vi "Add mppt data to log file.vi"(0 "Experiment Indicator":string, 1 "Cell details cluster":T3={"Cell Position"=16, "Cell Label"="", "Pixel to measure"=0, "Area (cm^2)"=0.126, "Variable"="", "Variable value"="", "Scan settings in queue"=0, "Light or dark"="", "Measurement Type"=""} {"Pixel to measure" items=["All", "1", "2", "3", "4", "5", "6", "7", "8"]}, 3 "Intensity (no. of suns)":string, 4 "mppt folder path":path, 5 "mppt file path":path, 7 "Scan settings":T1={"J-V scan"=TRUE, "J-t scan"=FALSE, "Min voltage (V)"=0.0, "Max voltage (V)"=1.4, "Step (V)"=0.01, "Measurement delay (ms)"=10.0, "1st scan FB-SC"=TRUE, "Inverted structure"=FALSE, "Stabilisation time (s)"=0.0, "Stabilisation mode"=0, "Stabilisation value (V or A) "=0.0, "Step time (s)"=1.0, "Integration time"=0, "Repeat light scans"=FALSE, "Stabilisation in the dark?"=FALSE, "J-t Min (V)"=0.0, "J-t Max (V)"=1.4, "J-t Step (V)"=0.01, "Max. power stabilisation"=FALSE, "J-t 1st scan FB-SC"=TRUE, "J-t Inverted structure"=FALSE, "Max power tracking"=FALSE, "Vmp (V)"=0.7, "Total stabilisation time (s)"=100.0, "J-t best pixel only"=0, "Max power best pixel only"=0, "Vmp from J-V scan"=FALSE, "Intensity dependence"=FALSE, "P dep best pixel only"=0, "External quantum efficiency"=FALSE, "EQE best pixel only"=0, "WL min (nm)"=300.0, "WL max (nm)"=900.0, "WL step (nm)"=5.0, "Wait (ms)"=100.0, "No. of repeat scans"=2.0, "Only repeat for best pixel"=0, "Chopper Freq.  (Hz)"=90.0, "Time Constant (s)"=2.0, "Stabilisation time step (s)"=1.0, "Illumination conditions"=2, "Scan rate min (V/s)"=0.1, "Scan rate max (V/s)"=1.0, "No. of scan rate steps"=1.0, "Scan rate voltage step priority"=FALSE, "Scan rate measurement delay priority"=FALSE, "J-t Illumination conditions"=0, "White bias  (no. of suns)"=200.0, "Max P stab. Specific voltage"=FALSE} {"J-t Illumination conditions" items=["Light only", "Dark only", "Light then dark", "Dark then light"]; "No. of scan rate steps" min=1.0 step=1.0; "Illumination conditions" items=["Light only", "Dark only", "Light then dark", "Dark then light", "Light then dark then light", "Dark then light then dark"]; "Time Constant (s)" items=["0.003", "0.01", "0.03", "0.1", "0.3", "1", "3", "10", "30", "100"]; "Only repeat for best pixel" items=["only for best pixel", "for best 2 pixels", "for best 3 pixels", "for best 4 pixels", "for best 5 pixels", "for best 6 pixels", "for best 7 pixels", "for all pixels"]; "No. of repeat scans" min=1.0 step=1.0; "EQE best pixel only" items=["only the best pixel", "the best 2 pixel", "the best 3 pixel", "the best 4 pixel", "the best 5 pixel", "the best 6 pixel", "the best 7 pixel", "all pixels"]; "P dep best pixel only" items=["only the best pixel", "the best 2 pixels", "the best 3 pixels", "the best 4 pixels", "the best 5 pixels", "the best 6 pixels", "the best 7 pixels", "all pixels"]; "Max power best pixel only" items=["only the best pixel", "the best 2 pixels", "the best 3 pixels", "the best 4 pixels", "the best 5 pixels", "the best 6 pixels", "the best 7 pixels", "all pixels"]; "J-t best pixel only" items=["only the best pixel", "the best 2 pixels", "the best 3 pixels", "the best 4 pixels", "the best 5 pixels", "the best 6 pixels", "the best 7 pixels", "all pixels"]; "Integration time" items=["Fast", "Normal", "High Accuracy"]; "Stabilisation mode" items=["V", "I"]; "Measurement delay (ms)" min=10.0}) -> (14 "Master Log":string[][](table), 15 "File path for master log":path)   [LabVIEW 2011]
uses:
  TypeDefs/Scan settings.ctl
  TypeDefs/Settings Boolean.ctl
  <vilib>/Utility/file.llb/Write To Spreadsheet File (string).vi
  <vilib>/Utility/file.llb/Read From Spreadsheet File (string).vi
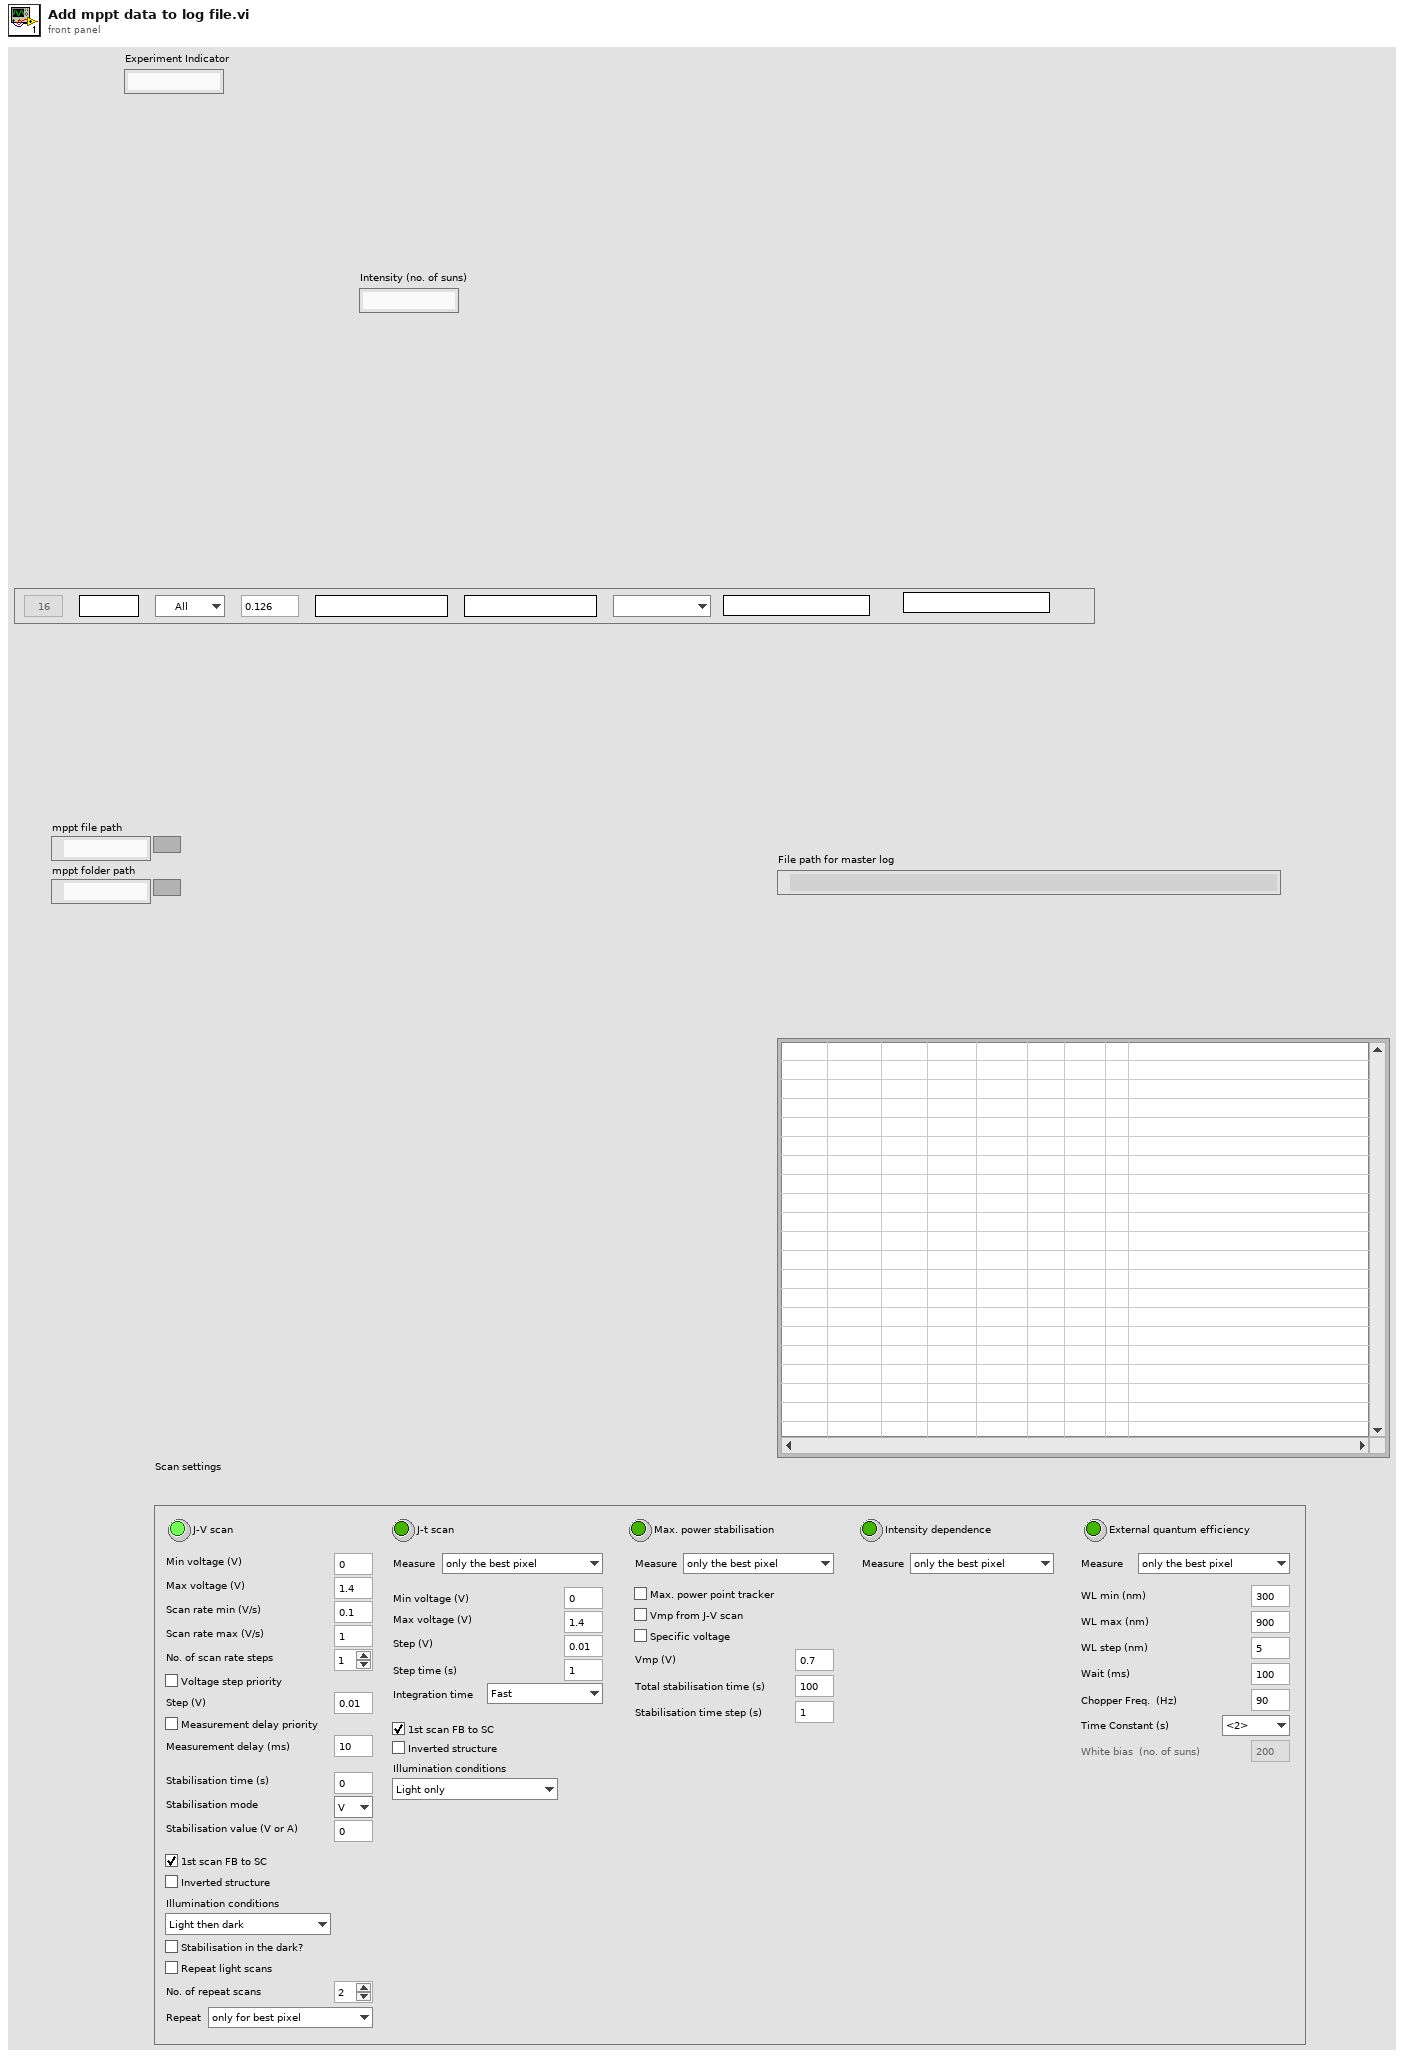
[diagram p1: front panel]
types:
  T1 = typedef "Scan settings.ctl" = cluster{"J-V scan":T2, "J-t scan":bool, "Min voltage (V)":dbl, "Max voltage (V)":dbl, "Step (V)":dbl, "Measurement delay (ms)":dbl, "1st scan FB-SC":bool, "Inverted structure":bool, "Stabilisation time (s)":dbl, "Stabilisation mode":u16, "Stabilisation value (V or A) ":dbl, "Step time (s)":dbl, "Integration time":u16, "Repeat light scans":bool, "Stabilisation in the dark?":bool, "J-t Min (V)":dbl, "J-t Max (V)":dbl, "J-t Step (V)":dbl, "Max. power stabilisation":bool, "J-t 1st scan FB-SC":bool, "J-t Inverted structure":bool, "Max power tracking":bool, "Vmp (V)":dbl, "Total stabilisation time (s)":dbl, "J-t best pixel only":u16, "Max power best pixel only":u16, "Vmp from J-V scan":bool, "Intensity dependence":bool, "P dep best pixel only":u16, "External quantum efficiency":bool, "EQE best pixel only":u16, "WL min (nm)":dbl, "WL max (nm)":dbl, "WL step (nm)":dbl, "Wait (ms)":dbl, "No. of repeat scans":dbl, "Only repeat for best pixel":u16, "Chopper Freq.  (Hz)":dbl, "Time Constant (s)":dbl, "Stabilisation time step (s)":dbl, "Illumination conditions":u16, "Scan rate min (V/s)":dbl, "Scan rate max (V/s)":dbl, "No. of scan rate steps":dbl, "Scan rate voltage step priority":bool, "Scan rate measurement delay priority":bool, "J-t Illumination conditions":u16, "White bias  (no. of suns)":dbl, "Max P stab. Specific voltage":bool}
  T2 = typedef "Settings Boolean.ctl" = bool
  T3 = cluster{"Cell Position":i32, "Cell Label":string, "Pixel to measure":u16, "Area (cm^2)":dbl, "Variable":string, "Variable value":string, "Scan settings in queue":u16, "Light or dark":string, "Measurement Type":string}
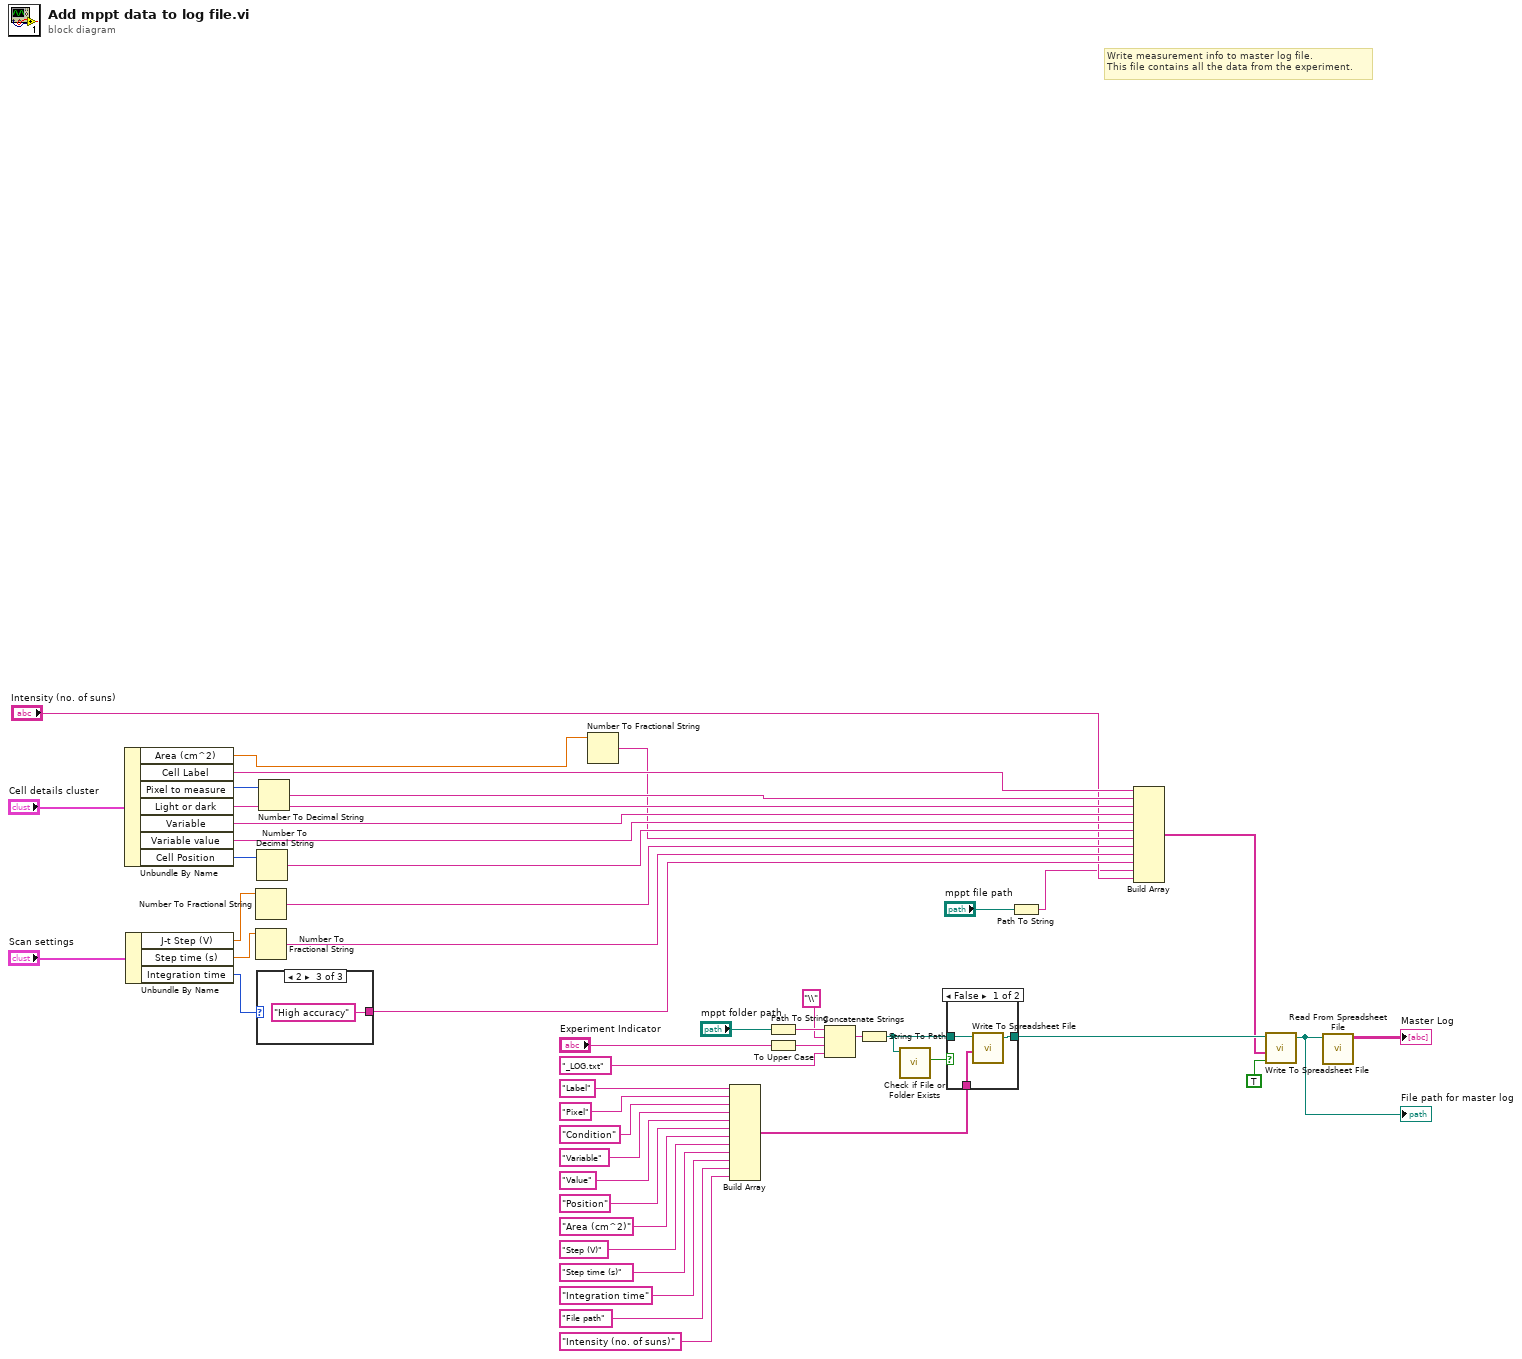
[diagram p0: block diagram]
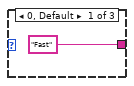
[diagram p2: hidden frame]
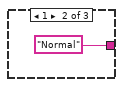
[diagram p3: hidden frame]
diagram:
  # "Write measurement info to master log file.\nThis file contains all the data from the experiment."
  n1 = Unbundle By Name("Cell details cluster") -> ("Area (cm^2)"=w12:dbl, "Cell Label"=w19:string, "Pixel to measure"=w47:u16, "Light or dark"=w17:string, "Variable"=w16:string, "Variable value"=w15:string, "Cell Position"=w14:i32)
  n2 = Unbundle By Name("Scan settings") -> ("J-t Step (V)"=w20:dbl, "Step time (s)"=w10:dbl, "Integration time"=w21:u16)
  n3 = Number To Fractional String(number=w20) -> (F-format string=w9:string)  [unwired: 3 in]
  n4 = Number To Fractional String(number=w10) -> (F-format string=w8:string)  [unwired: 3 in]
  n5 = Number To Decimal String(number=w14) -> (decimal integer string=w13:string)  [unwired: 1 in]
  n6 = case shown="2" w21 {
    tunnel: ["Fast" "Normal" "High accuracy"] -> w7
    frame 0, Default {
    }
    frame 1 {
    }
    frame 2 {
    }
  }
  n7 = Number To Decimal String(number=w47) -> (decimal integer string=w18:string)  [unwired: 1 in]
  n8 = Number To Fractional String(number=w12) -> (F-format string=w11:string)  [unwired: 3 in]
  n9 = Build Array("Label", "Pixel", "Condition", "Variable", "Value", "Position", "Area (cm^2)", "Step (V)", "Step time (s)", "Integration time", "File path", "Intensity (no. of suns)") -> (w23:string[])
  n10 = Path To String(path="mppt folder path") -> (string=w46:string)
  n11 = To Upper Case(1:"Experiment Indicator") -> (0:w39:string)
  n12 = Concatenate Strings(w46, "\\", w39, "_LOG.txt") -> (w44:string)
  n13 = String To Path(string=w44) -> (path=w37:path)
  n14 = call <vilib>:"Check if File or Folder Exists.vi"("path"=w37) -> ("file or folder exists?"=w38:bool)  [unwired: 8 in, 2 out]
  n15 = case shown="False" w38 {
    tunnel: w37 -> [w54 w55]
    tunnel: [w53 w55] -> w36
    tunnel: w23 -> [w52 _]
    frame False {
      n16 = call-poly <vilib>:"Write To Spreadsheet File.vi"("1D data"=w52, "file path (dialog if empty)"=w54) -> ("new file path (Not A Path if cancelled)"=w53:path)  [unwired: 6 in]
    }
    frame True {
    }
  }
  n17 = Path To String(path="mppt file path") -> (string=w4:string)
  n18 = Build Array(w19, w18, w17, w16, w15, w13, w11, w9, w8, w7, w4, "Intensity (no. of suns)") -> (w5:string[])
  n19 = call-poly <vilib>:"Write To Spreadsheet File.vi"("append to file? (new file:F)"=TRUE, "1D data"=w5, "file path (dialog if empty)"=w36) -> ("new file path (Not A Path if cancelled)"=w41:path)  [unwired: 5 in]
  "File path for master log" <- w41
  n20 = call-poly <vilib>:"Read From Spreadsheet File.vi"("file path (dialog if empty)"=w41) -> ("all rows"=→"Master Log":string[][])  [unwired: 6 in, 4 out]
